vi "QueryExistingConnectingString.vi"(8 "error in (no error)":errorcluster, 10 "Unregister if Invalid?":bool=TRUE, 11 "Service":T1) -> (0 "error out":errorcluster, 2 "Connection String":string, 3 "MicronCLI out":refnum<class "MicronCLI.lvclass">)   [LabVIEW 2019, in "MicronClient.lvclass"]
uses:
  MicronClient.lvclass
  MicronCLI/Typedefs/ServiceDetails.ctl
  MicronCLI/MicronCLI.lvclass
  MicronCLI/Typedefs/Message.ctl
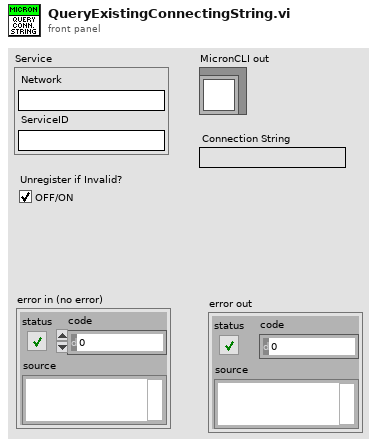
[diagram p1: front panel]
types:
  T1 = typedef "MicronCLI.lvclass/ServiceDetails.ctl" = cluster{"Network":string, "ServiceID":string}
  T2 = typedef "MicronCLI.lvclass/Message.ctl" = cluster{"Command":string, "Payload":string}
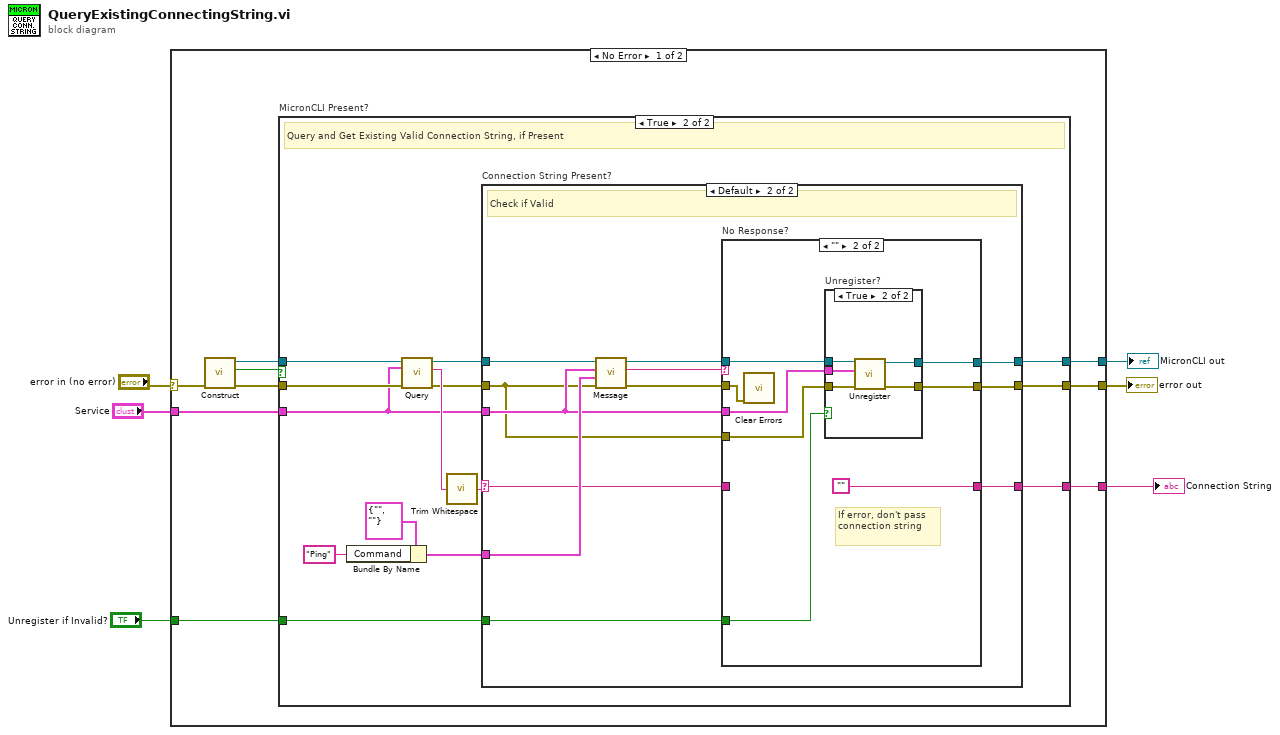
[diagram p0: block diagram]
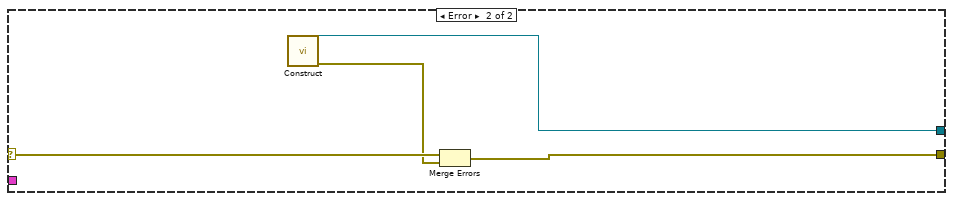
[diagram p6: hidden frame]
diagram:
  n1 = case shown="No Error" "error in (no error)" {
    selector: "error in (no error)" -> [w8 w67]
    tunnel: "Service" -> [w14 _]
    tunnel: [w13 w68] -> w5
    tunnel: [w12 _] -> w4
    tunnel: [w11 w65] -> w3
    tunnel: "Unregister if Invalid?" -> [w7 _]
    frame No Error {
      n2 = call "Construct.vi"("error in (no error)"=w8) -> ("error out"=w9:errorcluster, "Present?"=w15:bool, "MicronCLI out"=w10:refnum<class "MicronCLI.lvclass">)  [unwired: 8 in]
      n3 = case "MicronCLI Present?" shown="True" w15 {
        tunnel: w9 -> [w17 w30]
        tunnel: w10 -> [w16 w29]
        tunnel: [w17 w25] -> w11
        tunnel: [_ w24] -> w12
        tunnel: [w16 w23] -> w13
        tunnel: w14 -> [_ w19]
        tunnel: w7 -> [_ w18]
        frame False {
        }
        frame True {
          # "Query and Get Existing Valid Connection String, if Present"
          n4 = Bundle By Name(cluster=T2 {"Command"="", "Payload"=""} ("Message"), "Command"="Ping") -> (w20:T2)
          n5 = call-dynamic "Query.vi"("error in (no error)"=w30, "Service"=w19, "MicronCLI in"=w29) -> ("error out"=w28:errorcluster, "ConnectionString"=w31:string, "MicronCLI out"=w27:refnum<class "MicronCLI.lvclass">)  [unwired: 6 in]
          n6 = call <vilib>:"Trim Whitespace.vi"("string"=w31) -> ("trimmed string"=w26:string)  [unwired: 1 in]
          n7 = case "Connection String Present?" shown="Default" w26 {
            selector: w26 -> [w33 w37]
            tunnel: w28 -> [w34 w39]
            tunnel: w27 -> [w32 w46]
            tunnel: w19 -> [_ w41]
            tunnel: [w34 w44] -> w25
            tunnel: [w33 w40] -> w24
            tunnel: [w32 w42] -> w23
            tunnel: w20 -> [_ w45]
            tunnel: w18 -> [_ w35]
            frame "" {
            }
            frame Default {
              # "Check if Valid"
              n8 = call-dynamic "Message.vi"("error in (no error)"=w39, "Message"=w45, "Service"=w41, "MicronCLI in"=w46) -> ("error out"=w36:errorcluster, "Response"=w38:string, "MicronCLI out"=w43:refnum<class "MicronCLI.lvclass">)  [unwired: 5 in]
              n9 = case "No Response?" shown="\"\"" w38 {
                tunnel: [w47 w57] -> w44
                tunnel: w43 -> [w49 w56]
                tunnel: [w49 w55] -> w42
                tunnel: w41 -> [_ w54]
                tunnel: [w48 ""] -> w40
                tunnel: w39 -> [_ w52]
                tunnel: w37 -> [w48 _]
                tunnel: w36 -> [w47 w51]
                tunnel: w35 -> [_ w50]
                frame Default {
                  # "Valid Response"
                }
                frame "" {
                  # "If error, don't pass connection string"
                  n10 = call <vilib>:"Clear Errors.vi"("error in (no error)"=w51) -> ()  [unwired: 5 in, 2 out]
                  n11 = case "Unregister?" shown="True" w50 {
                    tunnel: [w58 w64] -> w57
                    tunnel: w56 -> [w59 w63]
                    tunnel: [w59 w62] -> w55
                    tunnel: w54 -> [_ w61]
                    tunnel: w52 -> [w58 w60]
                    frame False {
                    }
                    frame True {
                      n12 = call-dynamic "Unregister.vi"("error in (no error)"=w60, "Service"=w61, "MicronCLI in"=w63) -> ("error out"=w64:errorcluster, "MicronCLI out"=w62:refnum<class "MicronCLI.lvclass">)  [unwired: 7 in]
                    }
                  }
                }
              }
            }
          }
        }
      }
    }
    frame Error {
      n13 = call "Construct.vi"() -> ("error out"=w66:errorcluster, "MicronCLI out"=w68:refnum<class "MicronCLI.lvclass">)  [unwired: 9 in, 1 out]
      n14 = Merge Errors(w67, w66) -> (w65:errorcluster)
    }
  }
  "MicronCLI out" <- w5
  "Connection String" <- w4
  "error out" <- w3
